vi "Filter Interfaces.vi"(7 "Interfaces":refnum<class "Interface Documenation.lvclass">[](array[class]), 8 "error in (no error)":errorcluster {"code" format="Error %.0f"}, 11 "VIDoc Printer In":refnum<class "VIDoc Printer.lvclass">) -> (0 "error out":errorcluster {"code" format="Error %.0f"}, 3 "VIDoc Printer Out":refnum<class "VIDoc Printer.lvclass">, 5 "Filtered Interfaces":refnum<class "Interface Documenation.lvclass">[](array[class]))   [LabVIEW 2023, in "VIDoc Printer.lvlib" / "VIDoc Printer.lvclass"]
uses:
  VIDoc Printer.lvclass
  Parsing/Interface Documenation/Interface Documenation.lvclass
  VIDoc Printer.lvclass/VIDoc Printer.ctl
  Parsing/Interface Documenation/Interface Documenation.lvclass/Interface Documenation.ctl
  Parsing/Interface Documenation/Get Interface Info.vi
  Accessors/Get Library Scope.vi
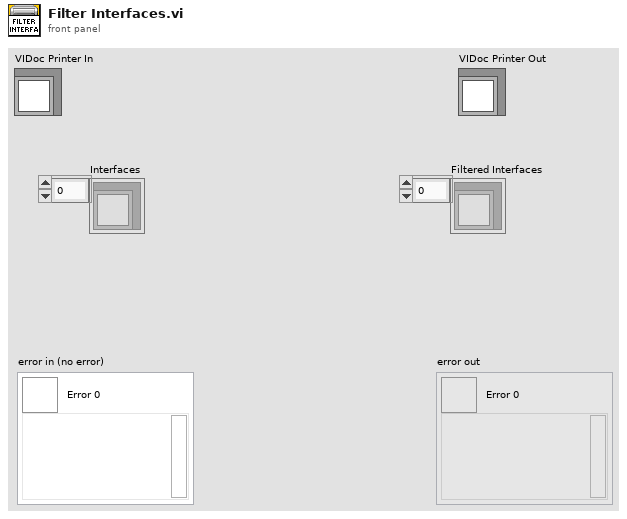
[diagram p1: front panel]
types:
  T1 = cluster{"Public":bool, "Community":bool, "Private":bool, "Unknown":bool}
  T2 = typedef "VIDoc Parsing.lvlib/Base Class Info Cluster.ctl" = cluster{"Name":string, "Icon":T3, "Version":cluster{"Major":u16, "Minor":u16, "Fix":u16, "Build":u16}, "Description":string, "Friends":string[], "ChildRefsRestricted":bool, "TransferMustOverrides":bool, "Path":path, "Qualified Name":string, "Class Scope":enum32{"invalid scope", "public", "private", "protected", "community"}}
  T3 = typedef "imagedata.ctl" = cluster{"image type":i32, "image depth":i32, "image":u8[], "mask":u8[], "colors":u32[], "Rectangle":cluster{"left":i16, "top":i16, "right":i16, "bottom":i16}}
  T4 = enum32{"invalid scope", "public", "private", "protected", "community"}
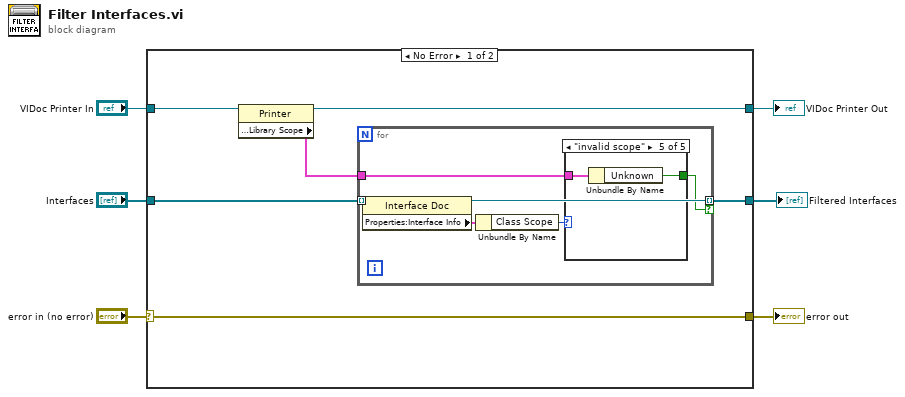
[diagram p0: block diagram]
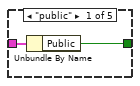
[diagram p2: hidden frame]
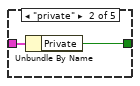
[diagram p3: hidden frame]
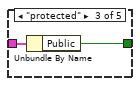
[diagram p4: hidden frame]
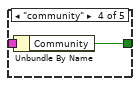
[diagram p5: hidden frame]
diagram:
  n1 = case shown="No Error" "error in (no error)" {
    selector: "error in (no error)" -> [w11 w31]
    tunnel: [w11 w31] -> w5
    tunnel: [w10 w30] -> w3
    tunnel: "VIDoc Printer In" -> [w12 w30]
    tunnel: "Interfaces" -> [w9 w29]
    tunnel: [w7 w29] -> w1
    frame No Error {
      n2 = property class="Printer"(reference=w12) -> (reference out=w10:refnum<class "VIDoc Printer.lvclass">, "Properties:Settings:Library Scope:Library Scope"=w8:T1)  [unwired: 1 in, 1 out]
      n3 = for {
        tunnel: w9 -> [w18] mode=indexing
        tunnel: w8 -> [w15]
        tunnel: [w14] -> w7 mode=indexing if=w13
        n4 = property class="Interface Doc"(reference=w18) -> (reference out=w14:refnum<class "Interface Documenation.lvclass">, "Properties:Interface Info"=w17:T2)  [unwired: 1 in, 1 out]
        n5 = Unbundle By Name(w17) -> ("Class Scope"=w16:T4)
        n6 = case shown="\"invalid scope\"" w16 {
          tunnel: w15 -> [w20 w22 w24 w26 w28]
          tunnel: [w19 w21 w23 w25 w27] -> w13
          frame "public" {
            n7 = Unbundle By Name(w20) -> ("Public"=w19:bool)
          }
          frame "private" {
            n8 = Unbundle By Name(w22) -> ("Private"=w21:bool)
          }
          frame "protected" {
            n9 = Unbundle By Name(w24) -> ("Public"=w23:bool)
          }
          frame "community" {
            n10 = Unbundle By Name(w26) -> ("Community"=w25:bool)
          }
          frame "invalid scope" {
            n11 = Unbundle By Name(w28) -> ("Unknown"=w27:bool)
          }
        }
      }
    }
    frame Error {
    }
  }
  "error out" <- w5
  "VIDoc Printer Out" <- w3
  "Filtered Interfaces" <- w1
